vi "channel operation tests.vi"() -> (0 "error out":errorcluster, 1 "size(s) 2":i32, 2 "size(s)":i32, 3 "channels match":bool)   [LabVIEW 2013, in "tag select module tests.lvlib"]
uses:
  tag select module tests.lvlib
  module/configuration/tag select module configuration.lvclass
  <vilib>/NI/Tag Bus/tag/tag descriptor.lvclass/tag descriptor.ctl
  <vilib>/NI/Tag Bus/tag/read tag name.vi
  <vilib>/NI/Tag Bus Module Framework/channel/TBM channel.lvclass
panel:
  out "Array 2":string[](array[string])
  out "Array":string[](array[string])
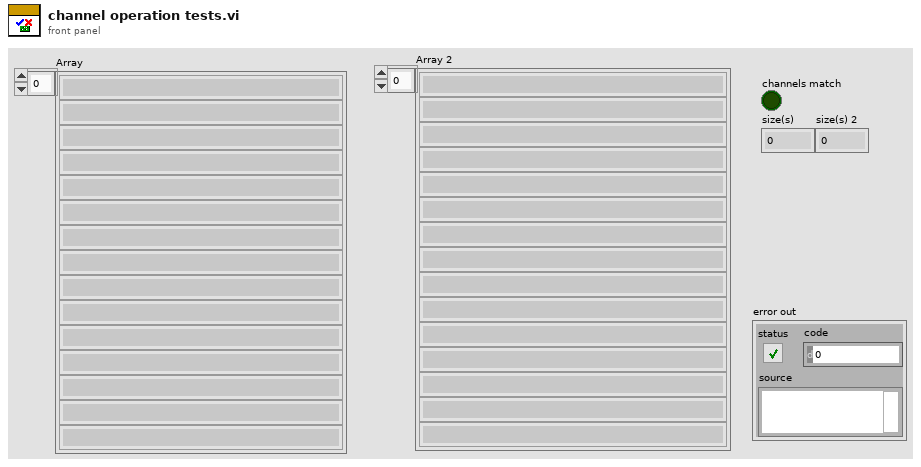
[diagram p1: front panel]
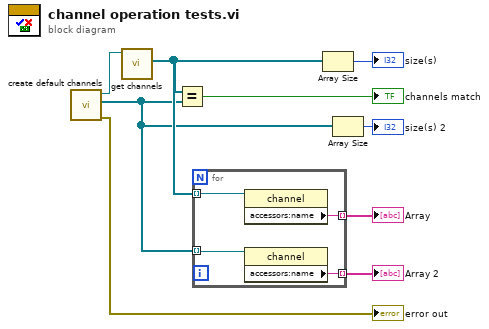
[diagram p0: block diagram]
diagram:
  n1 = call "create default channels.vi"() -> ("error out"=→"error out":errorcluster, "channels"=w2:refnum<class "TBM channel.lvclass">[], "module"=w8:refnum<class "tag select module configuration.lvclass">)  [unwired: 8 in, 1 out]
  n2 = call-dynamic "get channels.vi"("tag select module configuration in"=w8) -> ("channels"=w4:refnum<class "TBM channel.lvclass">[])  [unwired: 9 in, 1 out]
  n3 = Equal?(x=w4, y=w2) -> (x = y?=→"channels match":bool)
  n4 = for {
    tunnel: w4 -> [w13] mode=indexing
    tunnel: [w12] -> w3 mode=indexing
    tunnel: w2 -> [w11] mode=indexing
    tunnel: [w10] -> w1 mode=indexing
    n5 = property class="channel"(reference=w13) -> ("accessors:name"=w12:string)  [unwired: 1 in, 2 out]
    n6 = property class="channel"(reference=w11) -> ("accessors:name"=w10:string)  [unwired: 1 in, 2 out]
  }
  "Array" <- w3
  "Array 2" <- w1
  n7 = Array Size(array=w4) -> (size(s)=→"size(s)":i32)
  n8 = Array Size(array=w2) -> (size(s)=→"size(s) 2":i32)
